vi "BulbSender.vi"() -> ()   [LabVIEW 2020]
uses:
  <vilib>/httpClient/PUTBuffer.vi
  <vilib>/httpClient/LabVIEWHTTPClient.lvlib
panel:
  in  "Cluster":cluster{"Boolean":bool}
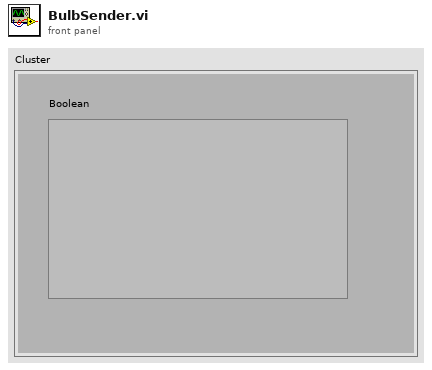
[diagram p1: front panel]
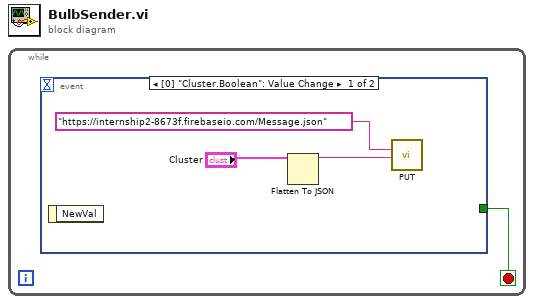
[diagram p0: block diagram]
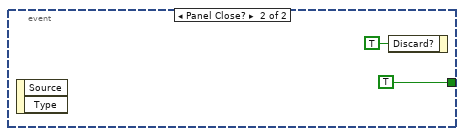
[diagram p2: hidden frame]
diagram:
  n1 = while {
    stop <- w1 stop-if-true
    n2 = event shown="[0] \"Cluster.Boolean\": Value Change" {
      selector: _ -> [_ _]
      dyn-events: _ -> [_ _]
      timeout: _ -> [_ _]
      tunnel: [_ TRUE] -> w1
      event "Cluster.Boolean": Value Change {
        n3 = event-data() -> ()  [unwired: 1 in, 1 out]
        n4 = Flatten To JSON(anything="Cluster") -> (JSON string=w2:string)  [unwired: 2 in, 1 out]
        n5 = call-poly <vilib>:"PUT.vi"("url"="https://internship2-8673f.firebaseio.com/Message.json", "buffer"=w2) -> ()  [unwired: 10 in, 4 out]
      }
      event Panel Close? {
        n6 = event-data() -> ()  [unwired: 1 in, 2 out]
        n7 = event-data("Discard?"=TRUE) -> ()  [unwired: 1 in, 1 out]
      }
    }
  }
